vi "Validate.vi"(8 "error in (no error)":errorcluster, 10 "Hardware Configuration":T1={"Stage Configuration"={"Serial Port"="COM3", "Forward Step (mm)"=0.4, "Lane Length (mm)"=6.0, "Lane Separation (mm)"=0.8, "Stage Type"=enum."Disabled", "Autofocus Z Planes"=9, "Autofocus Range (um)"=30.0, "Stage Limits"={"Y Min"=-4.5, "Y Max"=3.0, "X Min"=-19.0, "X Max"=33.5}, "Slide (mm)"={"top"=-22300.0, "right"=-13000.0, "width"=60000.0, "height"=25400.0}}, "Microscope Configuration"={"Serial Port"="COM2", "Microscope Type"=enum."TE2000", "Detection Settings"=[]}, "Virtual Camera Configuration"={"Camera Type"=enum."Hamamatsu"}, "Laser Configuration"=[], "Installed Cameras"=[], "Power Meter Configuration"={"Power Meter Type"=enum."Disabled", "attenuation"=53.2, "instrument handle"="USB0::0x1313::0x8075::P5001392::INSTR"}, "DAQ Configuration"={"Shutters"=[], "fluidics trigger line"="Dev1/port1/line1", "camera trigger line"="", "COM Port"="COM3", "Device type"=enum."NI DAQ"}}, 11 "Protocol in":refnum<class "Protocol.lvclass">) -> (0 "error out":errorcluster, 2 "Ok?":bool, 3 "Protocol out":refnum<class "Protocol.lvclass">)   [LabVIEW 2023, in "Automation.lvlib" / "Protocol.lvclass"]
uses:
  Protocol.lvclass
  Resources/Type Defs/Hardware Configuration.ctl
  Resources/Type Defs/Stage Configuration.ctl
  Resources/Type Defs/Microscope Configuration.ctl
  Resources/Type Defs/Microscope Type.ctl
  Resources/Type Defs/Virtual Camera Configuration.ctl
  Resources/Type Defs/Camera Type.ctl
  Resources/Type Defs/Laser Configuration.ctl
  Resources/Type Defs/Physical Camera Assignment.ctl
  Resources/Type Defs/DAQ Configuration.ctl
  Resources/Type Defs/Shutter Configuration.ctl
  Resources/Type Defs/Sync Device Type.ctl
  Resources/Type Defs/Movie auto-numbering.ctl
  Protocol.lvclass/Protocol.ctl
  Hardware/NI DAQ/NI DAQ.lvlib
  Application/Application.lvlib
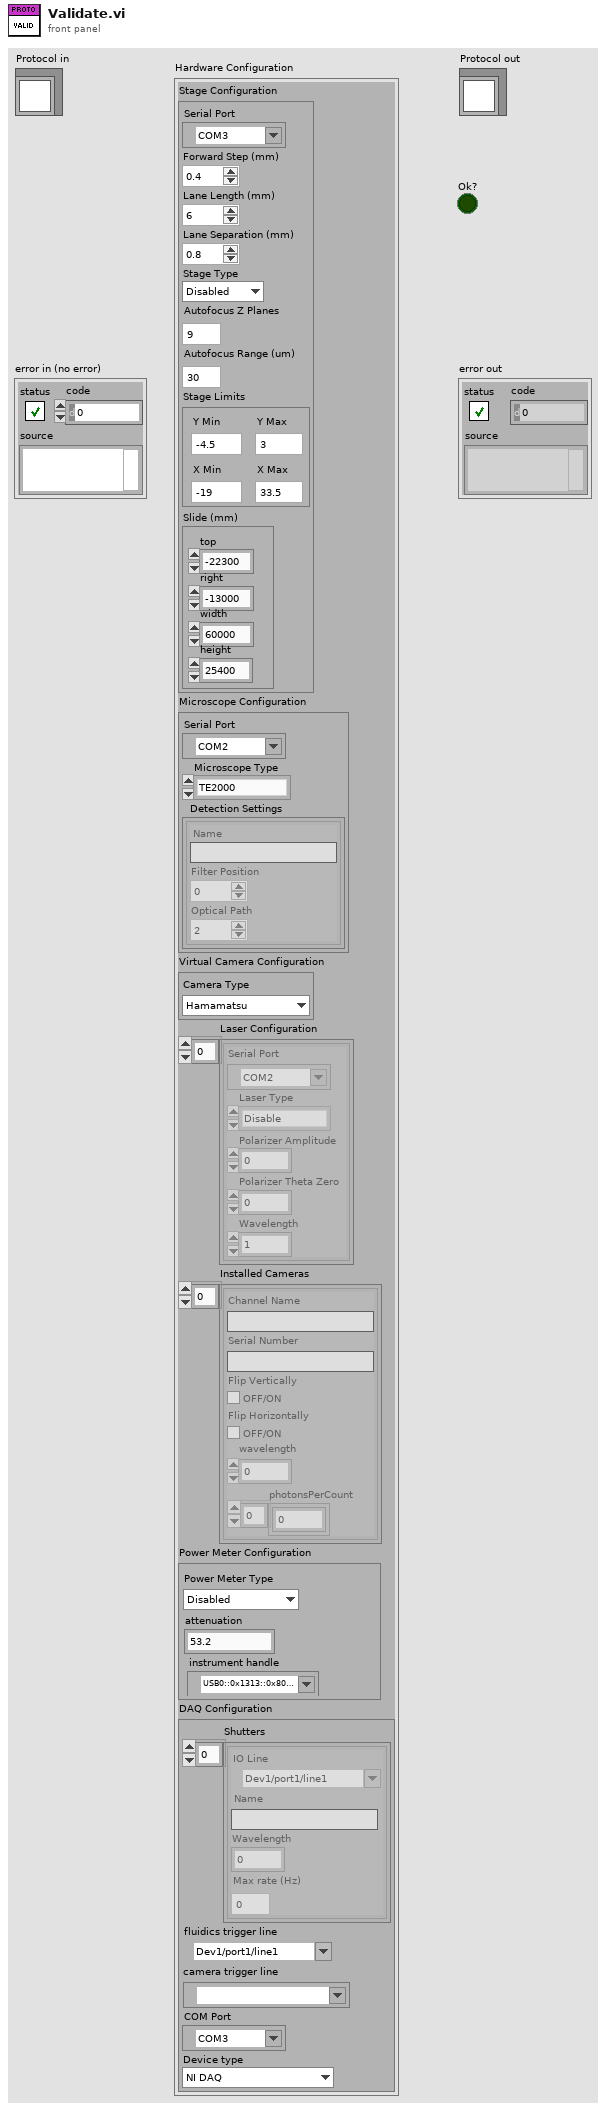
[diagram p1: front panel]
types:
  T1 = typedef "Hardware Configuration.ctl" = cluster{"Stage Configuration":T2, "Microscope Configuration":T3, "Virtual Camera Configuration":T5, "Laser Configuration":T7[], "Installed Cameras":T8[], "Power Meter Configuration":cluster{"Power Meter Type":enum16{"Disabled", "Thorlabs", "Newport", "Coherent"}, "attenuation":dbl, "instrument handle":refnum<visa-resource-name>}, "DAQ Configuration":T9}
  T2 = typedef "Stage Configuration.ctl" = cluster{"Serial Port":refnum<visa-resource-name>, "Forward Step (mm)":dbl, "Lane Length (mm)":dbl, "Lane Separation (mm)":dbl, "Stage Type":enum16{"Disabled", "ESP301", "Ti2", "Ludl", "ASI", "Simulate"}, "Autofocus Z Planes":i32, "Autofocus Range (um)":dbl, "Stage Limits":cluster{"Y Min":dbl, "Y Max":dbl, "X Min":dbl, "X Max":dbl}, "Slide (mm)":cluster{"top":dbl, "right":dbl, "width":dbl, "height":dbl}}
  T3 = typedef "Microscope Configuration.ctl" = cluster{"Serial Port":refnum<visa-resource-name>, "Microscope Type":T4, "Detection Settings":cluster{"Name":string, "Filter Position":u16, "Optical Path":u16}[]}
  T4 = typedef "Microscope Type.ctl" = enum16{"Disable", "TE2000", "Eclipse Ti", "Ti2"}
  T5 = typedef "Virtual Camera Configuration.ctl" = cluster{"Camera Type":T6}
  T6 = typedef "Camera Type.ctl" = enum16{"Hamamatsu", "Andor", "Photometrics"}
  T7 = typedef "Laser Configuration.ctl" = cluster{"Serial Port":refnum<visa-resource-name>, "Laser Type":enum16{"Disable", "Laser Quantum", "Coherent OBIS", "PRM1-Z8", "Coherent HOPS", "Cobolt"}, "Polarizer Amplitude":dbl, "Polarizer Theta Zero":dbl, "Wavelength":u16}
  T8 = typedef "Physical Camera Assignment.ctl" = cluster{"Channel Name":string, "Serial Number":string, "Flip Vertically":bool, "Flip Horizontally":bool, "wavelength":i16, "photonsPerCount":dbl[]}
  T9 = typedef "DAQ Configuration.ctl" = cluster{"Shutters":T10[], "fluidics trigger line":tag, "camera trigger line":tag, "COM Port":refnum<visa-resource-name>, "Device type":T11}
  T10 = typedef "Shutter Configuration.ctl" = cluster{"IO Line":tag, "Name":string, "Wavelength":u16, "Max rate (Hz)":dbl}
  T11 = typedef "Sync Device Type.ctl" = enum16{"Disabled", "NI DAQ", "Arduino DAQ", "Microsync"}
  T12 = typedef "Movie auto-numbering.ctl" = enum16{"Single movie", "Movie series", "Multi-lane series", "Sweep Parameter"}
  T13 = typedef "Camera Settings.ctl" = cluster{"Exposure Time (ms)":dbl, "Binning":enum16{"1x1", "2x2", "4x4"}, "Scan Mode":i32, "Frames to Acquire":dbl, "Pixel Correction":bool, "Frames to Skip":u32, "File Path":path, "Duty cycle":dbl, "ALEX":bool, "Shutter Enable":bool[], "fluidics trigger, ms (0=disabled)":dbl, "Bit Depth":u16, "Image Width (px)":u16, "Image Height (px)":u16, "Horizontal Offset (px)":u16, "Vertical Offset (px)":u16}
  T14 = typedef "Param Sweep.ctl" = cluster{"Parameter":enum16{"Laser Power (mW)", "Exposure Time (ms)"}, "Values":u32[]}
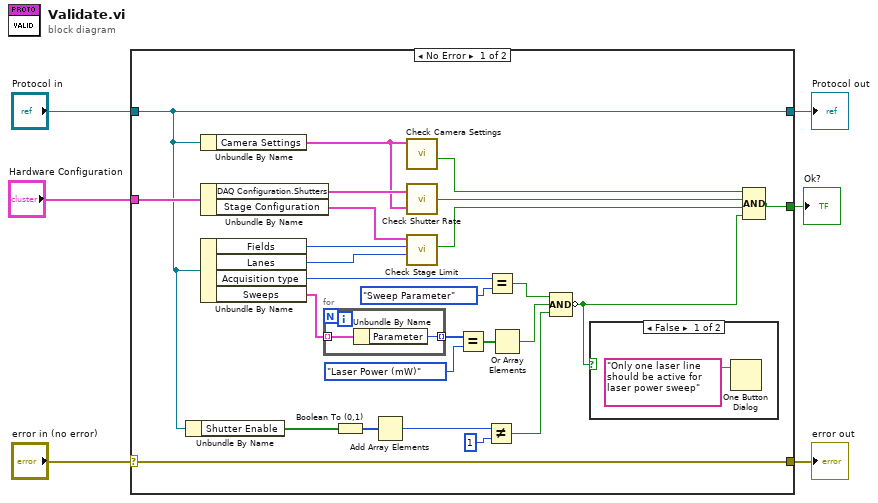
[diagram p0: block diagram]
diagram:
  n1 = case shown="No Error" "error in (no error)" {
    selector: "error in (no error)" -> [w32 w37]
    tunnel: [w32 w37] -> w5
    tunnel: [w17 w36] -> w3
    tunnel: "Protocol in" -> [w17 w36]
    tunnel: "Hardware Configuration" -> [w31 _]
    tunnel: [w26 _] -> w1
    frame No Error {
      n2 = Unbundle By Name(w17) -> ("Shutter Enable"=w16:bool[])
      n3 = Unbundle By Name(w17) -> ("Camera Settings"=w29:T13)
      n4 = Unbundle By Name(w31) -> ("DAQ Configuration.Shutters"=w30:T10[], "Stage Configuration"=w23:T2)
      n5 = Unbundle By Name(w17) -> ("Fields"=w25:i32, "Lanes"=w24:i32, "Acquisition type"=w21:T12, "Sweeps"=w11:T14[])
      n6 = for {
        tunnel: w11 -> [w34] mode=indexing
        tunnel: [w33] -> w9 mode=indexing
        n7 = Unbundle By Name(w34) -> ("Parameter"=w33:enum16{"Laser Power (mW)", "Exposure Time (ms)"})
      }
      n8 = Boolean To (0,1)(Boolean=w16) -> (0, 1=w15:i16[])
      n9 = Add Array Elements(numeric array=w15) -> (sum=w14:i16)
      n10 = call "Check Camera Settings.vi"("Camera Settings In"=w29) -> ("Ok"=w28:bool)  [unwired: 10 in]
      n11 = call "Check Shutter Rate.vi"("Camera Settings"=w29, "Shutters"=w30) -> ("OK?"=w27:bool)
      n12 = call "Check Stage Limit.vi"("Lanes"=w24, "Fields"=w25, "Stage Configuration"=w23) -> ("In Range?"=w22:bool)  [unwired: 8 in]
      n13 = Equal?(x=w9, y=enum16{"Laser Power (mW)", "Exposure Time (ms)"}."Laser Power (mW)") -> (x = y?=w7:bool[])
      n14 = Not Equal?(x=w14, y=i16 1) -> (x != y?=w12:bool)
      n15 = Equal?(x=w21, y=Movie_auto-numbering."Sweep Parameter") -> (x = y?=w19:bool)
      n16 = Or Array Elements(Boolean array=w7) -> (logical OR=w10:bool)
      n17 = Compound Arithmetic op=AND(w19, w10, w12) -> (invert w18:bool)
      n18 = case shown="False" w18 {
        frame False {
          n19 = One Button Dialog(message="Only one laser line should be active for laser power sweep") -> ()  [unwired: 1 in, 1 out]
        }
        frame True {
        }
      }
      n20 = Compound Arithmetic op=AND(w28, w27, w22, w18) -> (w26:bool)
    }
    frame Error {
    }
  }
  "error out" <- w5
  "Protocol out" <- w3
  "Ok?" <- w1
